vi "PI Dialog List GUI.vi"(6 "Select Item":i32=-1, 8 "error in (no error)":errorcluster, 10 "List Items":string[](array[string]), 11 "Prompt":string) -> (0 "error out":errorcluster, 1 "Index":i32=-1, 2 "Selected List Item":string, 3 "Cancelled?":bool)   [LabVIEW 2011]
uses:
  Keystroke.ctl
panel:
  in  "Cancel":bool caption="Add Field"
  in  "OK":bool caption="Add Field"
  in  "Listbox":i32(listbox)
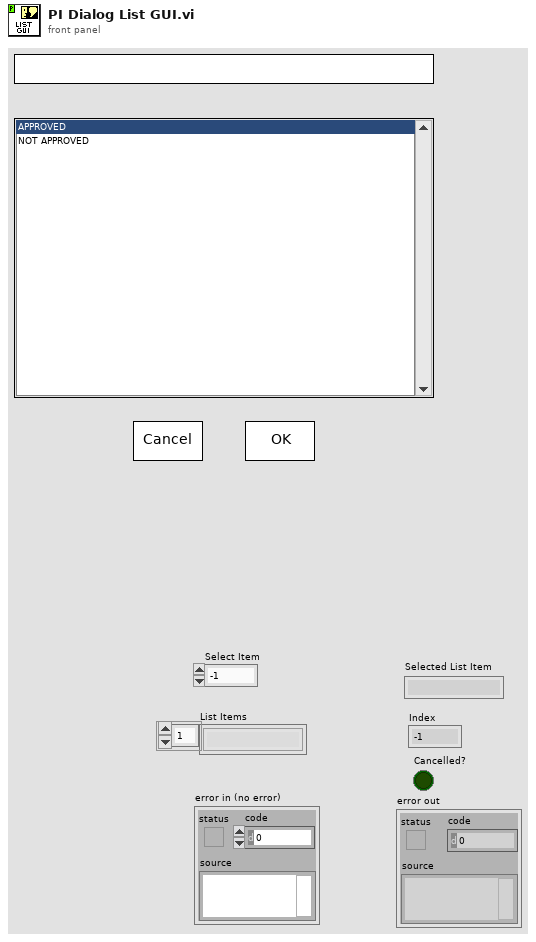
[diagram p1: front panel]
types:
  T1 = typedef "Keystroke.ctl" = enum16{"None", "CTRL+ALT+A", "CTRL+ALT+F", "CTRL+ALT+L", "CTRL+ALT+M", "CTRL+ALT+P", "CTRL+ALT+R"}
  T2 = typedef "eventvkey.ctl" = enum16{"ASCII", "Enter", "Return", "Shift", "Ctrl", "Alt", "Cmd", "Opt", "Caps", "NumLock", "Clear", "Break", "Up", "Down", "Left", "Right", "Insert", "Delete", "Home", "End", "PageUp", "PageDown", "Escape", "Help", "Pause", "ScrollLock", "F1", "F2", "F3", "F4", "F5", "F6", "F7", "F8", "F9", "F10", "F11", "F12", "F13", "F14", "F15", "F16", "F17", "F18", "F19", "F20", "F21", "F22", "F23", "F24", "Play", "VolumeUp", "VolumeDown", "Mute", "Two Byte Char"}
  T3 = cluster{"Shift":bool, "Ctrl":bool, "Alt":bool, "Cmd":bool, "Opt":bool}
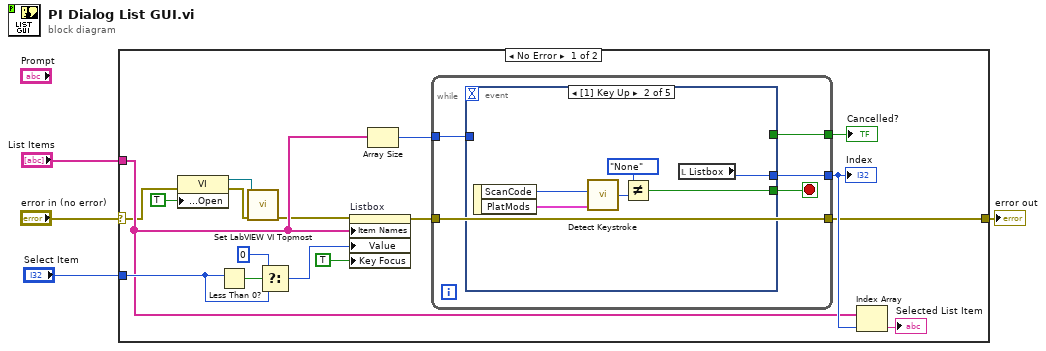
[diagram p0: block diagram]
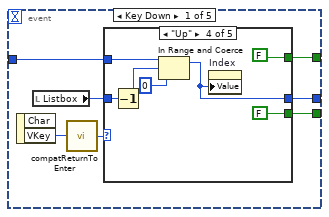
[diagram p2: hidden frame]
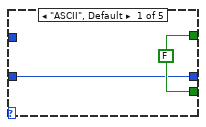
[diagram p3: hidden frame]
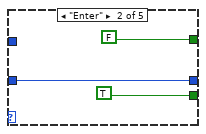
[diagram p4: hidden frame]
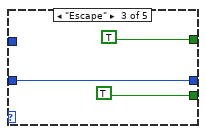
[diagram p5: hidden frame]
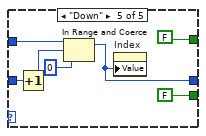
[diagram p6: hidden frame]
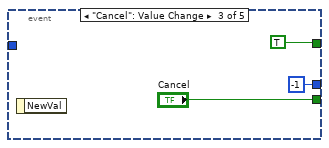
[diagram p7: hidden frame]
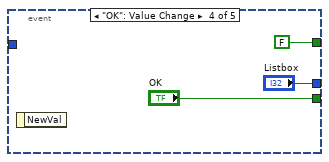
[diagram p8: hidden frame]
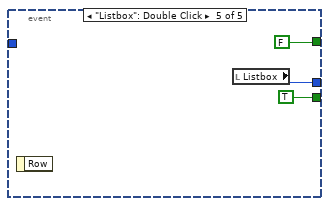
[diagram p9: hidden frame]
diagram:
  n1 = case shown="No Error" "error in (no error)" {
    selector: "error in (no error)" -> [w7 w71]
    tunnel: [w18 w71] -> w4
    tunnel: "List Items" -> [w12 _]
    tunnel: "Select Item" -> [w14 _]
    frame No Error {
      n2 = property class="VI"(error in=w7, "Front Panel Window:Open"=TRUE) -> (reference out=w9:refnum<vi>, error out=w6:errorcluster)  [unwired: 1 in]
      n3 = Less Than 0?(x=w14) -> (x < 0?=w16:bool)
      n4 = call "Set LabVIEW VI Topmost.vi"("error in (no error)"=w6, "VI Refnum (null)"=w9) -> ("error out"=w10:errorcluster)  [unwired: 7 in, 2 out]
      n5 = Select(t=0, s=w16, f=w14) -> (s? t:f=w13:i32)
      n6 = property on="Listbox" class="LstBox (strict)"(error in=w10, "Item Names"=w12, "Value"=w13, "Key Focus"=TRUE) -> (error out=w17:errorcluster)  [unwired: 1 in, 1 out]
      n7 = Array Size(array=w12) -> (size(s)=w11:i32)
      n8 = while {
        tunnel: w17 -> [w26]
        tunnel: [w26] -> w18
        tunnel: [w24] -> w19
        tunnel: [w23] -> w21
        tunnel: w11 -> [w22]
        stop <- w25 stop-if-true
        n9 = event shown="[1] Key Up" {
          selector: _ -> [_ _ _ _ _]
          dyn-events: _ -> [_ _ _ _ _]
          timeout: _ -> [_ _ _ _ _]
          tunnel: [w31 w57 "Cancel" "OK" TRUE ("cancel")] -> w25
          tunnel: [w29 w58 -1 ("Listbox") "Listbox" w70] -> w24
          tunnel: [w32 _ TRUE FALSE FALSE ("cancel")] -> w23
          tunnel: w22 -> [w28 _ _ _ _]
          event Key Down {
            n10 = event-data() -> ("VKey"=w27:T2)  [unwired: 2 out]
            n11 = local read "Listbox"() -> (w30:i32)
            n12 = call <vilib>:"compatReturnToEnter.vi"("VKey"=w27) -> ("VKey"=w33:T2)
            n13 = case shown="\"Up\"" w33 {
              tunnel: [w35 FALSE TRUE FALSE FALSE] -> w32
              tunnel: [w35 TRUE TRUE FALSE FALSE] -> w31
              tunnel: w30 -> [w34 w36 w39 w46 w53]
              tunnel: [w34 w36 w39 w42 w49] -> w29
              tunnel: w28 -> [_ _ _ w43 w50]
              frame "ASCII", Default {
                w35 = FALSE
              }
              frame "Enter" {
              }
              frame "Escape" {
              }
              frame "Up" {
                n14 = Decrement(x=w46) -> (x-1=w45:i32)
                n15 = In Range and Coerce(upper limit=w43, x=w45, lower limit=0) -> (coerced(x)=w42:i32)  [unwired: 1 out]
                n16 = property on="Index" class="DigNum (strict)"("Value"=w42) -> ()  [unwired: 2 in, 2 out]
              }
              frame "Down" {
                n17 = Increment(x=w53) -> (x+1=w52:i32)
                n18 = In Range and Coerce(upper limit=w50, x=w52, lower limit=0) -> (coerced(x)=w49:i32)  [unwired: 1 out]
                n19 = property on="Index" class="DigNum (strict)"("Value"=w49) -> ()  [unwired: 2 in, 2 out]
              }
            }
          }
          event Key Up {
            n20 = event-data() -> ("ScanCode"=w60:i16, "PlatMods"=w61:T3)  [unwired: 1 out]
            n21 = call "Detect Keystroke.vi"("PlatMods"=w61, "ScanCode"=w60) -> ("Keystroke"=w59:T1)  [unwired: 4 out]
            n22 = Not Equal?(x=Keystroke."None", y=w59) -> (x != y?=w57:bool)
            n23 = local read "Listbox"() -> (w58:i32)
          }
          event "Cancel": Value Change {
            n24 = event-data() -> ()  [unwired: 2 out]
          }
          event "OK": Value Change {
            n25 = event-data() -> ()  [unwired: 2 out]
          }
          event "Listbox": Double Click {
            n26 = event-data() -> ()  [unwired: 2 out]
            n27 = local read "Listbox"() -> (w70:i32)
          }
        }
      }
      "Index" <- w19
      "Cancelled?" <- w21
      n28 = Index Array(array=w12, index=w19) -> (element=→"Selected List Item":string)
    }
    frame Error {
    }
  }
  "error out" <- w4
